vi "GrowInfo.vi"(1 "XRef":refnum<vi>, 2 "State In":T5={"Input Type"=variant(dbl 0.0), "Width"=0, "Typedef Name"="", "Value Type"=variant, "Selection"=0, "Options"=[], "Selections"=[], "Display Selections"=[], "Element Names"=[], "Typedef Name Width"=0, "Display Selection Width"=[], "Code Generated"=FALSE, "Is DVR"=FALSE, "Write Lock"=FALSE}) -> (0 "Grow Info":T4)   [LabVIEW 2015, in "Read-Write-Signals.xnode"]
doc: "This ability VI is used to describe your XNode's grow behavior. GrowInfo is a cluster containing the following elements:\n Min Bounds: The minimum bounds of your XNode.\n Max Bounds: The maximum bounds of your XNode.\n Vertical Increment: The vertital grow increment of your XNode. Zero is interpreted as a one pixel increment.\n Horizontal Increment: The horizontal grow increment of your XNode. Zero is interpreted as a one pixel increment.\n Maintain Aspect?: Indicates that your XNode should maintain aspect ratio.\n Oval?: Indcates that your grow lines are drawn as an oval instead of a rectangle.\n Vertical Only Resize?: Indicates that your XNode only grows vertically.\n Horizontal Only Resize?: Indicates that your XNode only grows horizontally.\n Resize None?: Indicates that your XNode can not be resized.\n\nDefault behavior: Indicate that your XNode cannot be resized.\n\nThis ability does not provide UI and OS messages are not handled.\n\nSee also: OnResize"
uses:
  Read-Write-Signals.xnode
  State.ctl
  Read-Write-Signals Item.ctl
  Read-Write-Signals Sub Item.ctl
  Read-Write-Signals Sub Item Type.ctl
  Read-Write-Signals Selection.ctl
  Read-Write-Signals Display Selection.ctl
  <vilib>/XNodeSupport/XNodeBounds.ctl
  <vilib>/XNodeSupport/XNodeInt.ctl
  <vilib>/XNodeSupport/XNodeBool.ctl
  <vilib>/XNodeSupport/NI_XNodeSupport.lvlib
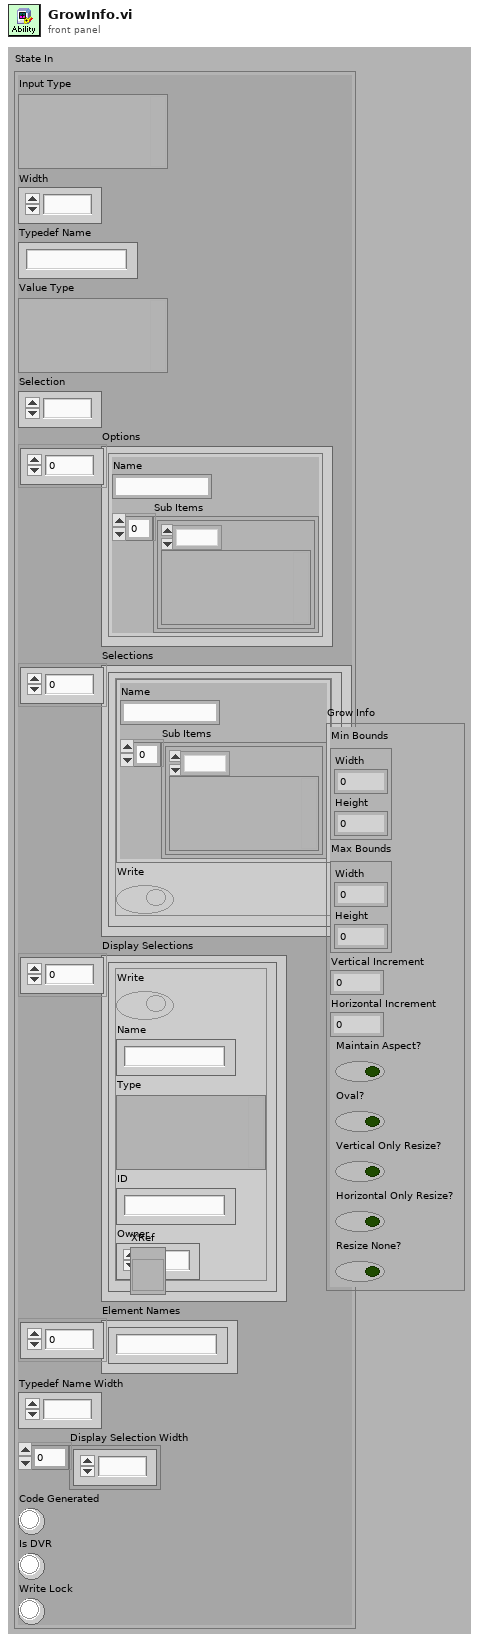
[diagram p1: front panel]
types:
  T1 = typedef "NI_XNodeSupport.lvlib/XNodeBounds.ctl" = cluster{"Width":T2, "Height":T2}
  T2 = typedef "NI_XNodeSupport.lvlib/XNodeInt.ctl" = i32
  T3 = typedef "NI_XNodeSupport.lvlib/XNodeBool.ctl" = bool
  T4 = cluster{"Min Bounds":T1, "Max Bounds":T1, "Vertical Increment":T2, "Horizontal Increment":T2, "Maintain Aspect?":T3, "Oval?":T3, "Vertical Only Resize?":T3, "Horizontal Only Resize?":T3, "Resize None?":T3}
  T5 = typedef "Read-Write-Signals.xnode/State.ctl" = cluster{"Input Type":variant, "Width":i32, "Typedef Name":string, "Value Type":variant, "Selection":i32, "Options":T6[], "Selections":T9[], "Display Selections":T10[], "Element Names":string[], "Typedef Name Width":i32, "Display Selection Width":i32[], "Code Generated":bool, "Is DVR":bool, "Write Lock":bool}
  T6 = typedef "Read-Write-Signals Item.ctl" = cluster{"Name":string, "Sub Items":T7[]}
  T7 = typedef "Read-Write-Signals Sub Item.ctl" = cluster{"Type":T8, "Value":variant}
  T8 = typedef "Read-Write-Signals Sub Item Type.ctl" = enum8{"Cluster Element", "Array Element", "Subarray"}
  T9 = typedef "Read-Write-Signals Selection.ctl" = cluster{"Item":T6, "Write":bool}
  T10 = typedef "Read-Write-Signals Display Selection.ctl" = cluster{"Write":bool, "Name":string, "Type":variant, "ID":string, "Owner":i32}
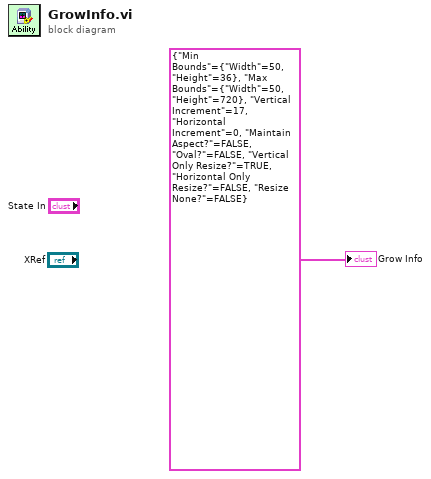
[diagram p0: block diagram]
diagram:
  "Grow Info" <- T4 {"Min Bounds"={"Width"=50, "Height"=36}, "Max Bounds"={"Width"=50, "Height"=720}, "Vertical Increment"=17, "Horizontal Increment"=0, "Maintain Aspect?"=FALSE, "Oval?"=FALSE, "Vertical Only Resize?"=TRUE, "Horizontal Only Resize?"=FALSE, "Resize None?"=FALSE} ("Grow Info")
